vi "Update Mode.vi"   [LabVIEW 2014, in "SLSC configuration Shared.lvlib"]
doc: "Updates the mode of the pins."
uses:
  SLSC configuration Shared.lvlib
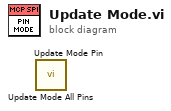
[diagram p0: block diagram]
diagram:
  n1 = call "Update Mode All Pins.vi"() -> ()  [unwired: 9 in, 3 out]
  n2 = call "Update Mode Pin.vi"() -> ()  [unwired: 9 in, 3 out]
